vi "MovemotorMengXYMain.vi"(6 "Joystick axis":i32, 8 "error in (no error)":errorcluster, 9 "XorYMAX":sgl, 10 "XorYMIN":sgl, 11 "Automation Refnum in":refnum<k7>) -> (0 "error out":errorcluster, 2 "Automation Refnum out":refnum<k7>, 3 "XorYPosition":sgl)   [LabVIEW 2014]
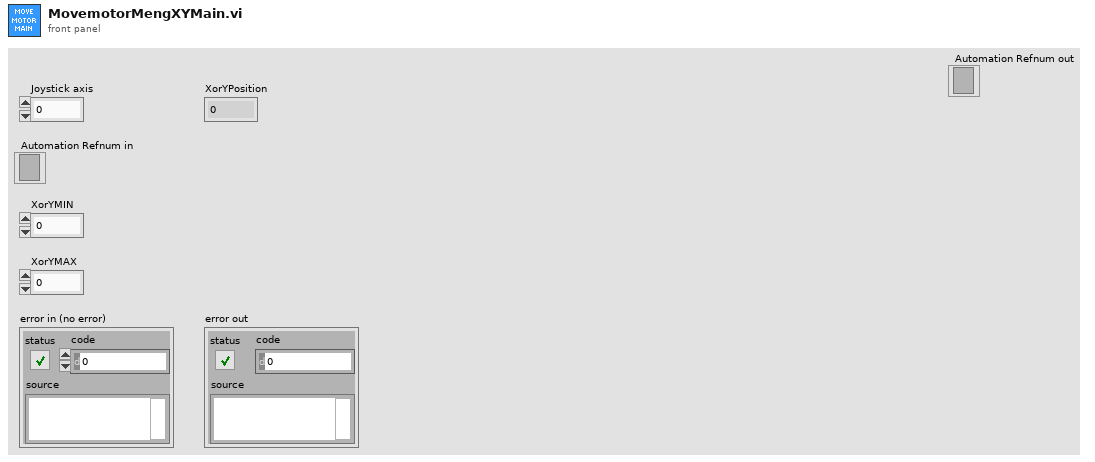
[diagram p1: front panel]
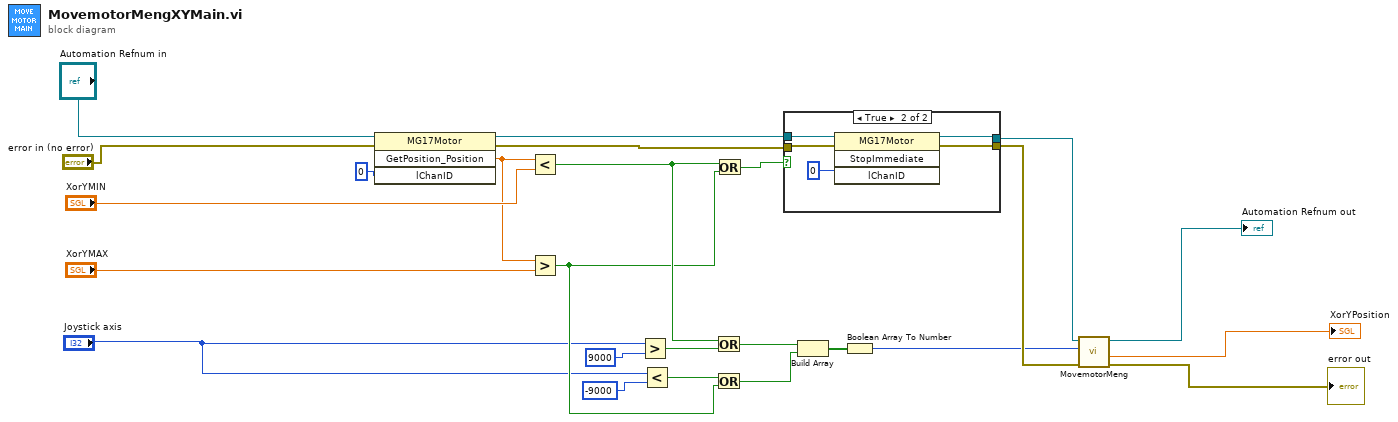
[diagram p0: block diagram]
diagram:
  n1 = invoke class="MG17Motor" method="GetPosition_Position"(reference="Automation Refnum in", error in="error in (no error)", "lChanID"=0) -> (reference out=w21:refnum<k7>, error out=w20:errorcluster, "GetPosition_Position"=w10:sgl)  [unwired: 1 in, 1 out]
  n2 = Less?(x=w10, y="XorYMIN") -> (x < y?=w18:bool)
  n3 = Greater?(x=w10, y="XorYMAX") -> (0:w17:bool)
  n4 = Greater?(x="Joystick axis", y=9000) -> (0:w12:bool)
  n5 = Less?(x="Joystick axis", y=-9000) -> (x < y?=w9:bool)
  n6 = Or(x=w18, y=w12) -> (x .or. y?=w13:bool)
  n7 = Or(x=w9, y=w17) -> (x .or. y?=w14:bool)
  n8 = Or(x=w18, y=w17) -> (x .or. y?=w19:bool)
  n9 = case shown="True" w19 {
    tunnel: w21 -> [w27 w32]
    tunnel: w20 -> [w26 w31]
    tunnel: [w26 w30] -> w23
    tunnel: [w27 w29] -> w22
    frame False {
    }
    frame True {
      n10 = invoke class="MG17Motor" method="StopImmediate"(reference=w32, error in=w31, "lChanID"=0) -> (reference out=w29:refnum<k7>, error out=w30:errorcluster)  [unwired: 1 in, 2 out]
    }
  }
  n11 = Build Array(w13, w14) -> (w4:bool[])
  n12 = Boolean Array To Number(Boolean array=w4) -> (number=w6:u32)
  n13 = call "MovemotorMeng.vi"("error in (no error)"=w23, "Numeric"=w6, "Automation Refnum in"=w22) -> ("error out"=→"error out":errorcluster, "Position"=→"XorYPosition":sgl, "Automation Refnum out"=→"Automation Refnum out":refnum<k7>)  [unwired: 6 in]
